vi "Refresh Listbox Changes.vi"(8 "error in":errorcluster, 10 "Only Show Changes (T)":bool=TRUE, 11 "Refresh Listbox":T2={"Item Names"=[], "Item Symbols"=[enum."Blank", enum."Incoming", enum."Outgoing", enum."Frame", enum."Signal", enum."Cluster"], "Change Flag"=[]}) -> (0 "error out":errorcluster, 2 "Item Symbols":T1[](array[typedef])=[enum."Blank", enum."Incoming", enum."Outgoing", enum."Frame", enum."Signal", enum."Cluster"], 3 "Item Names":string[][](array[string]))   [LabVIEW 2020, in "Communication Bus Template System Explorer.lvlib" / "Implementation.lvlib"]
doc: "This VI runs when the Add Port run-time menu is chosen. It allows the user to create a port with an associated database."
uses:
  Implementation.lvlib
  Types/Refresh Listbox.ctl
  Types/Refresh Symbols.ctl
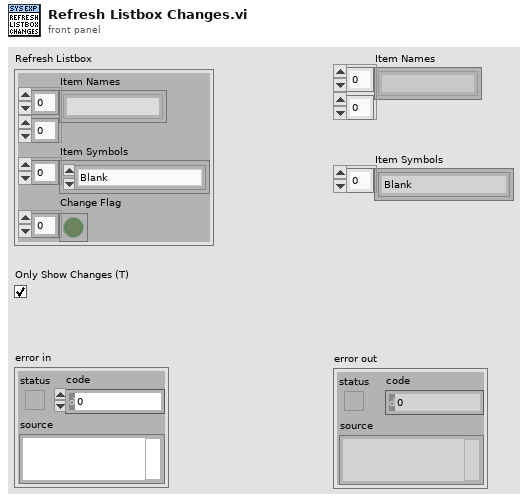
[diagram p1: front panel]
types:
  T1 = typedef "Communication Bus Template System Explorer.lvlib/Implementation.lvlib/Refresh Symbols.ctl" = enum16{"Blank", "Port", "Incoming", "Outgoing", "Frame", "Signal", "Cluster", "Baud Rate"}
  T2 = typedef "Communication Bus Template System Explorer.lvlib/Implementation.lvlib/Refresh Listbox.ctl" = cluster{"Item Names":string[][], "Item Symbols":T1[], "Change Flag":bool[]}
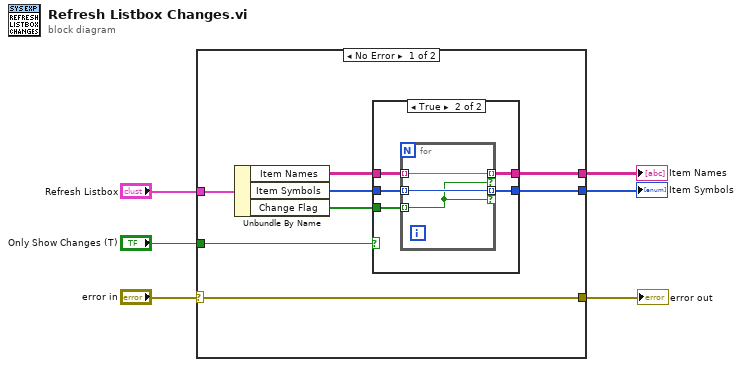
[diagram p0: block diagram]
diagram:
  n1 = case shown="No Error" "error in" {
    selector: "error in" -> [w7 w25]
    tunnel: "Refresh Listbox" -> [w11 _]
    tunnel: "Only Show Changes (T)" -> [w10 _]
    tunnel: [w9 _] -> w4
    tunnel: [w8 _] -> w3
    tunnel: [w7 w25] -> w1
    frame No Error {
      n2 = Unbundle By Name(w11) -> ("Item Names"=w14:string[][], "Item Symbols"=w13:T1[], "Change Flag"=w12:bool[])
      n3 = case shown="True" w10 {
        tunnel: w14 -> [w16 w21]
        tunnel: w13 -> [w15 w20]
        tunnel: w12 -> [_ w19]
        tunnel: [w16 w18] -> w9
        tunnel: [w15 w17] -> w8
        frame False {
        }
        frame True {
          n4 = for {
            tunnel: w21 -> [w24] mode=indexing
            tunnel: w20 -> [w23] mode=indexing
            tunnel: w19 -> [w22] mode=indexing
            tunnel: [w24] -> w18 mode=indexing if=w22
            tunnel: [w23] -> w17 mode=indexing if=w22
          }
        }
      }
    }
    frame Error {
    }
  }
  "error out" <- w1
  "Item Names" <- w4
  "Item Symbols" <- w3
